vi "FR_LED.vi"() -> ()   [LabVIEW 2014]
doc: "FR_LED\nvers. 8.6\nMiusra di Fotoresistenza vs I_LED"
uses:
  <vilib>/Utility/file.llb/Write To Spreadsheet File (DBL).vi
panel:
  in  "Fondo Scala CB33":dbl(ring)=10.0 items=["10"=10.0, "5"=5.0, "0.5"=0.5, "0.05"=0.05]
  in  "Fondo Scala CB68":dbl(ring)=10.0 items=["10"=10.0, "5"=5.0, "0.5"=0.5, "0.05"=0.05]
  in  "R_foto (kOhm)":dbl=10.0 format="%_4g"
  in  "R_LED (kOhm)":dbl=0.47 format="%_4g"
  in  "SALVA I DATI SU FILE":bool=TRUE caption="ON\nOFF"
  out "I_LED (mA)":dbl=0.8888888888888888 format="%_3g"
  out "No Misura":i32
  out "grafico FR-Iled":cluster{dbl[], dbl[]}(graph)={[0.0, 0.1111111111111111, 0.2222222222222222, 0.3333333333333333, 0.4444444444444444, 0.5555555555555556, 0.6666666666666666, 0.7777777777777777, 0.8888888888888888, 1.0], [-0.0004529765695386318, -0.014427021987432244, -0.01732511658045662, -0.018398951136659965, -0.018677776799501833, -0.019850837395018833, -0.020255658836403193, -0.020491458287726416, -0.020572059261143347, -0.020695232078207736]}
  out "Vin":dbl=0.8888888888888888 format="%_3g"
  out "FR (kOhm)":dbl=-0.020257183823893847 format="%_3f"
  in  "Nmis":i16=20
  in  "Vmax (V)":dbl=1.0 min=-10.0 max=10.0 step=0.1
  in  "Vmin (V)":dbl min=-10.0 max=10.0 step=0.1
  # "1) Scegliere il fondo scala dei canali di ingresso"
  # "Collegare il CB22 al LED.\nCollegare il CB33 alla fotoresistenza\nCollegare il CB68 alla resistenza in serie al LED.\nLa terra del circuito DEVE essere in comune alla terra della scheda  (CB29)."
  # "2) Selezionare il valore minimo e massimo della tensione di ingresso ed il numero di valori (equispaziati  tra gli estremi),  il valore della resistenza in serie al LED e il valore della resistenza in serie alla fotoresistenza."
  # "3) Premere la freccia bianca"
  # "Durante la misura gli indicatori mostrano i valori di Vin e Vout ed il numero progressivo della misura"
  # "Sul grafico viene mostrata la resistenza FR della fotocella in funzione della corrente che scorre nel LED"
  # "NO\nSI"
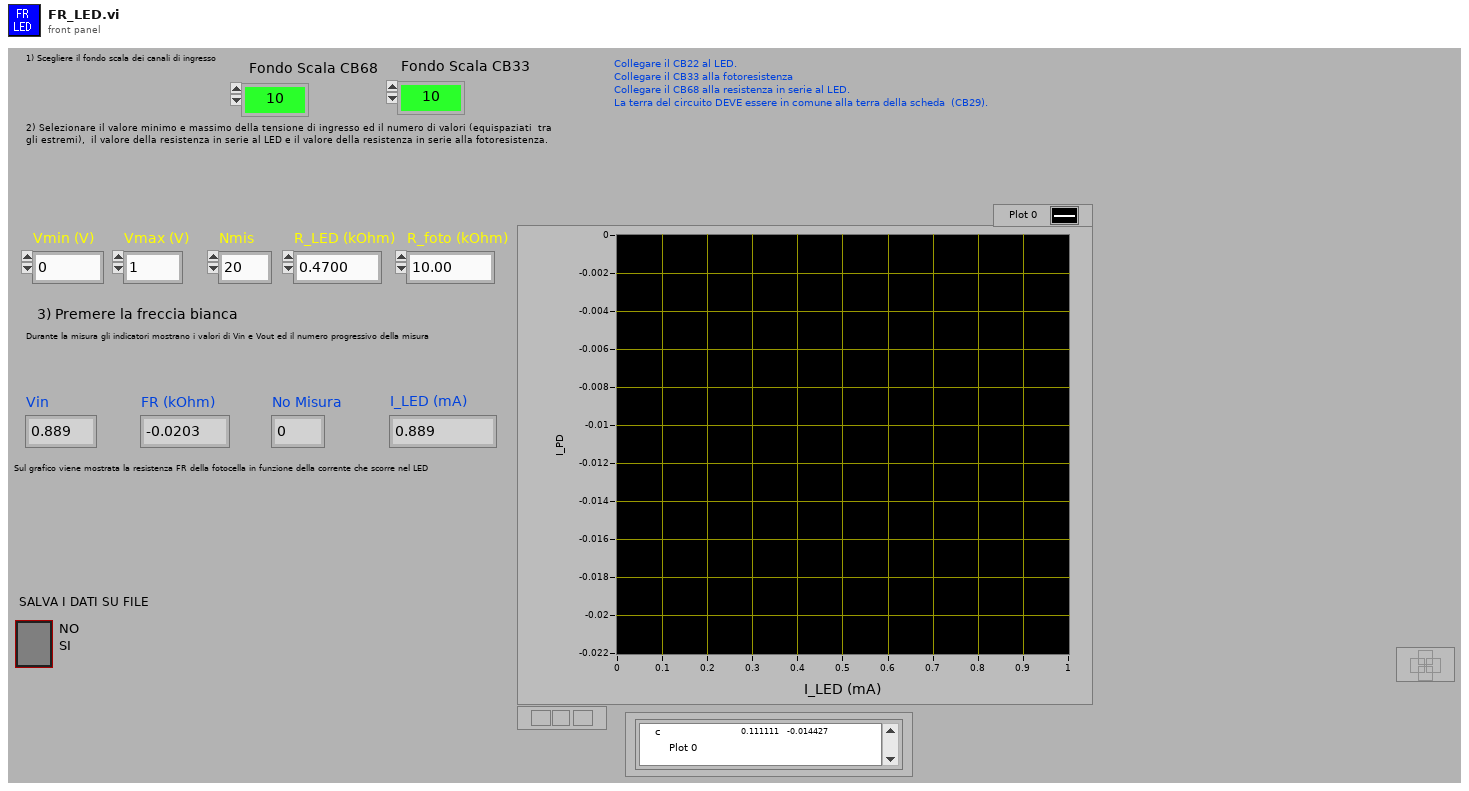
[diagram p1: front panel]
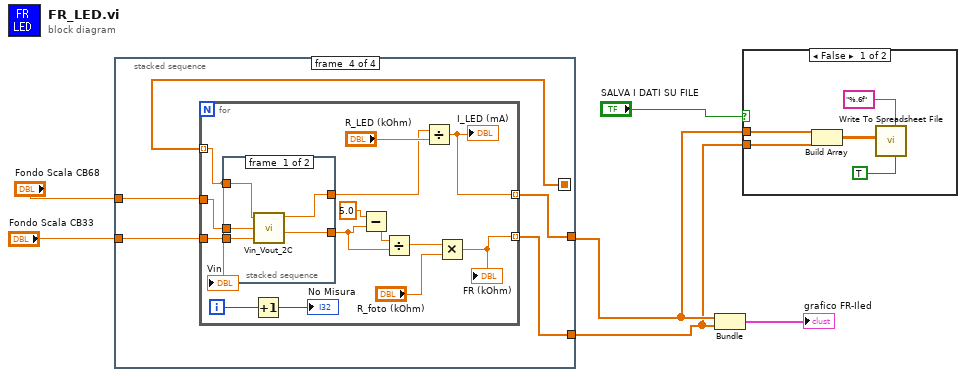
[diagram p0: block diagram]
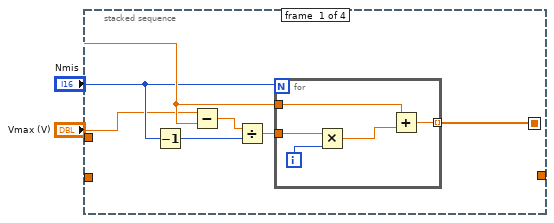
[diagram p3: hidden frame]
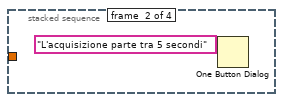
[diagram p4: hidden frame]
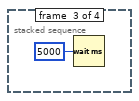
[diagram p5: hidden frame]
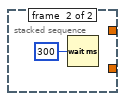
[diagram p6: hidden frame]
diagram:
  n1 = stacked-sequence {
    seq-local: [w9 _ _ _] -> [_ _ _ w24]
    tunnel: [_ _ _ w25] -> w3
    tunnel: [_ _ _ w23] -> w4
    tunnel: "Fondo Scala CB68" -> [_ _ _ w22]
    tunnel: "Fondo Scala CB33" -> [_ _ _ w21]
    frame #0 {
      n2 = Decrement(x="Nmis") -> (x-1=w12:i16)
      n3 = Subtract(x="Vmax (V)", y="Vmin (V)") -> (x-y=w13:dbl)
      n4 = Divide(x=w13, y=w12) -> (x/y=w11:dbl)
      n5 = for {
        N: "Nmis" -> [_]
        tunnel: "Vmin (V)" -> [w18]
        tunnel: [w17] -> w9 mode=indexing
        tunnel: w11 -> [w16]
        i -> [w15]
        n6 = Multiply(x=w16, y=w15) -> (x*y=w14:dbl)
        n7 = Add(x=w18, y=w14) -> (x+y=w17:dbl)
      }
    }
    frame #1 {
      n8 = One Button Dialog(message="L'acquisizione parte tra 5 secondi") -> ()  [unwired: 2 out]
    }
    frame #2 {
      n9 = Wait (ms)(milliseconds to wait=u32 5000) -> ()  [unwired: 1 out]
    }
    frame #3 {
      n10 = for {
        tunnel: w24 -> [w39] mode=indexing
        tunnel: [w28] -> w25 mode=indexing
        tunnel: [w34] -> w23 mode=indexing
        tunnel: w22 -> [w33]
        tunnel: w21 -> [w32]
        i -> [w38]
        n11 = stacked-sequence {
          tunnel: w39 -> [w44 _]
          tunnel: [w42 _] -> w29
          tunnel: [w43 _] -> w35
          tunnel: w33 -> [w41 _]
          tunnel: w32 -> [w40 _]
          frame #0 {
            n12 = call "Vin_Vout_2C.vi"("V in volt"=w44, "Fondo Scala AI0 (68)"=w41, "Fondo Scala AI1 (33)"=w40) -> ("V0 medio"=w43:dbl, "V1 medio"=w42:dbl)  [unwired: 2 out]
          }
          frame #1 {
            n13 = Wait (ms)(milliseconds to wait=u32 300) -> ()  [unwired: 1 out]
          }
        }
        n14 = Increment(x=w38) -> (x+1=→"No Misura":i32)
        n15 = Subtract(x=5.0, y=w29) -> (x-y=w30:dbl)
        n16 = Divide(x=w30, y=w29) -> (x/y=w27:dbl)
        n17 = Divide(x=w35, y="R_LED (kOhm)") -> (x/y=w34:dbl)
        "I_LED (mA)" <- w34
        n18 = Multiply(x=w27, y="R_foto (kOhm)") -> (x*y=w28:dbl)
        "FR (kOhm)" <- w28
        "Vin" <- w39
      }
    }
  }
  n19 = Bundle(w4, w3) -> (→"grafico FR-Iled":cluster{dbl[], dbl[]})  [unwired: 1 out]
  n20 = case shown="False" "SALVA I DATI SU FILE" {
    tunnel: w4 -> [w48 _]
    tunnel: w3 -> [w47 _]
    frame False {
      n21 = Build Array(w48, w47) -> (w49:dbl[][])
      n22 = call-poly <vilib>:"Write To Spreadsheet File.vi"("transpose? (no:F)"=TRUE, "format (%.3f)"="%.6f", "2D data"=w49) -> ()  [unwired: 3 in, 3 out]
    }
    frame True {
    }
  }
